vi "Write.vi"(8 "error in (no error)":errorcluster, 10 "Value":T1, 11 "Double Float.lvclass_340760 in":refnum<class "Var_I8.lvclass">) -> (0 "error out":errorcluster, 3 "Double Float.lvclass_340760 out":refnum<class "Var_I8.lvclass">)   [LabVIEW 2021, in "Var_I8.lvclass"]
uses:
  Var_I8.lvclass
  Type.ctl
  Var_I8.lvclass/Var_I8.ctl
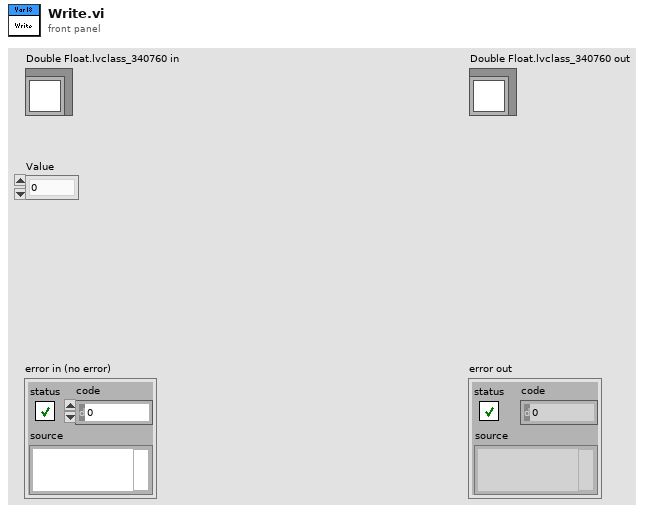
[diagram p1: front panel]
types:
  T1 = typedef "Var_I8.lvclass/Type.ctl" = i8
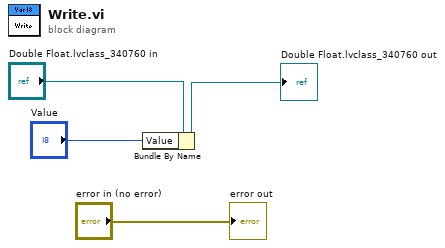
[diagram p0: block diagram]
diagram:
  n1 = Bundle By Name(cluster="Double Float.lvclass_340760 in", "Value"="Value") -> (→"Double Float.lvclass_340760 out":refnum<class "Var_I8.lvclass">)
  "error out" <- "error in (no error)"
